vi "Flatten.vi"(8 "error in (no error)":errorcluster, 11 "DAQ Digital Code Scan in":refnum<class "DAQ Digital Code Scan.lvclass">) -> (0 "error out":errorcluster, 3 "DAQ Digital Code Scan out":refnum<class "DAQ Digital Code Scan.lvclass">)   [LabVIEW 2012, in "DAQ Digital Code Scan.lvclass"]
uses:
  DAQ Digital Code Scan.lvclass
  Scanner/Scanner.lvclass
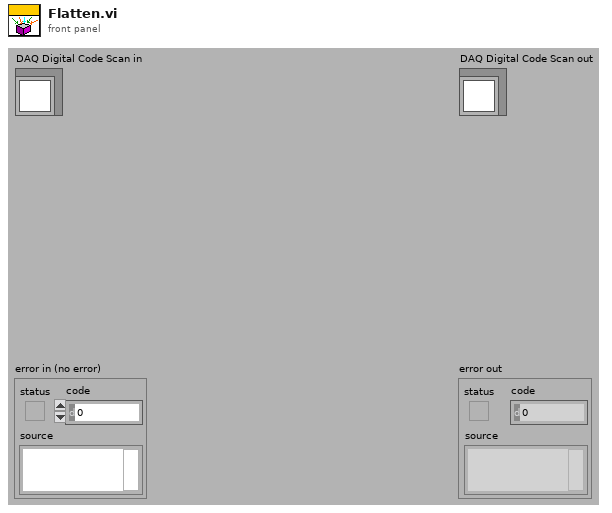
[diagram p1: front panel]
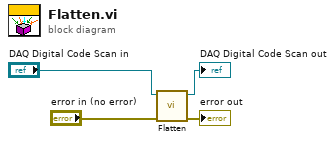
[diagram p0: block diagram]
diagram:
  n1 = call-parent "Flatten.vi"("error in (no error)"="error in (no error)", "Scanner in"="DAQ Digital Code Scan in") -> ("error out"=→"error out":errorcluster, "Scanner out"=→"DAQ Digital Code Scan out":refnum<class "DAQ Digital Code Scan.lvclass">)  [unwired: 8 in]
